vi "GetInstrumentInformation.vi"(8 "error in (no error)":errorcluster, 11 "RoomAlert in":refnum<class "RoomAlert.lvclass">) -> (0 "error out":errorcluster, 2 "Model IDs":string[][][](array[string]), 3 "RoomAlert out":refnum<class "RoomAlert.lvclass">)   [LabVIEW 2018, in "SensorPlugins.lvlib" / "RoomAlert.lvclass"]
doc: "Extracts the model name of the RoomAlert Instrument and also used to double check the connection to the instrument."
uses:
  RoomAlert.lvclass
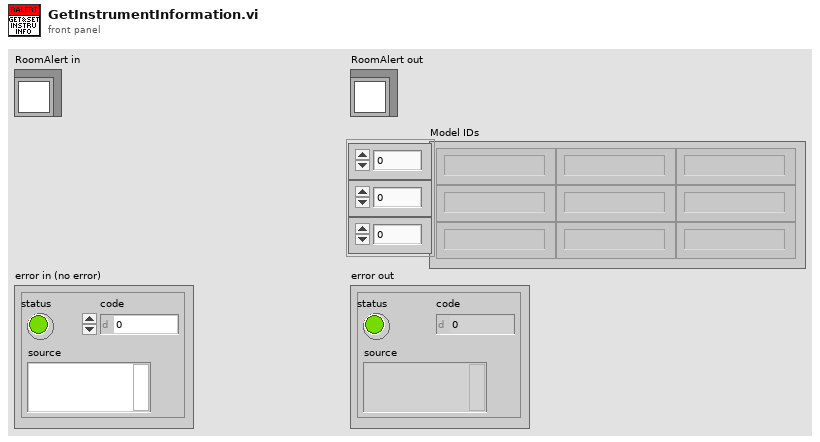
[diagram p1: front panel]
types:
  T1 = typedef "SensorPlugins.lvlib/RoomAlert.lvclass/RoomAlertControls.ctl" = cluster{"Connected?":bool, "IP Address of SNMP Device":string, "Port (161)":u16, "Community Name":string, "Measurements To Read Array":u16[], "Update LightTower?":bool, "LightTower":cluster{"Red":bool, "Amber":bool, "Green":bool, "Audio":bool}, "RoomAlert Model ID":string, "Sensor OID Numbers":string[][], "Sensor Light Tower OID Numbers":string[][]}[]
  T2 = typedef "SensorPlugins.lvlib/RoomAlert.lvclass/CommunicationControls.ctl" = refnum<k16>[]
  T3 = typedef "SensorPlugins.lvlib/RoomAlert.lvclass/MeasurementControls.ctl" = cluster{"Measurement RefreshTime (ms)":u32, "Measurement Name":string, "Timeout(ms)":i32, "Amber Warning Light Configuration":cluster{"Warning Temperture (Degrees C)":dbl, "Temperature Delta (Degrees C/Minute)":dbl, "Time Window (Minutes)":dbl}}
  T4 = cluster{"Connected?":bool, "IP Address of SNMP Device":string, "Port (161)":u16, "Community Name":string, "Measurements To Read Array":u16[], "Update LightTower?":bool, "LightTower":cluster{"Red":bool, "Amber":bool, "Green":bool, "Audio":bool}, "RoomAlert Model ID":string, "Sensor OID Numbers":string[][], "Sensor Light Tower OID Numbers":string[][]}
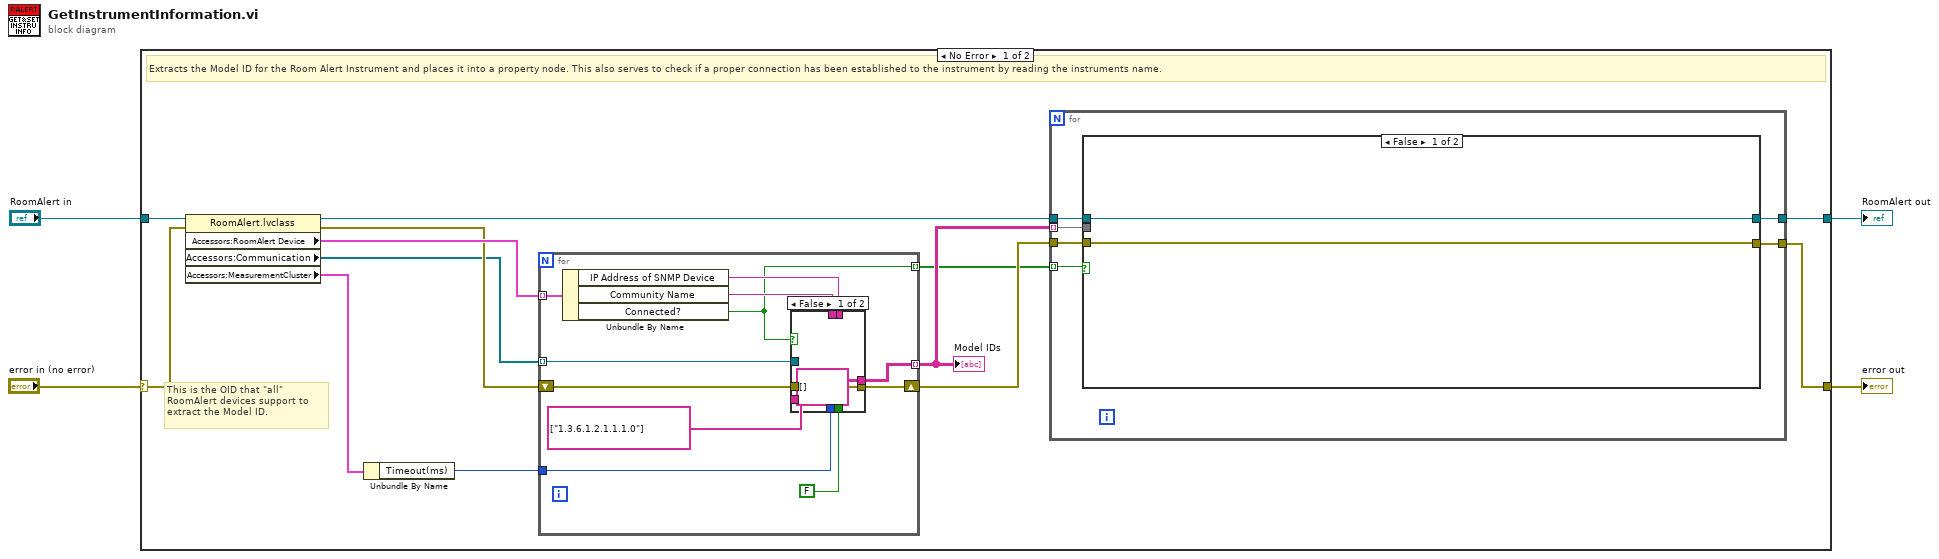
[diagram p0: block diagram]
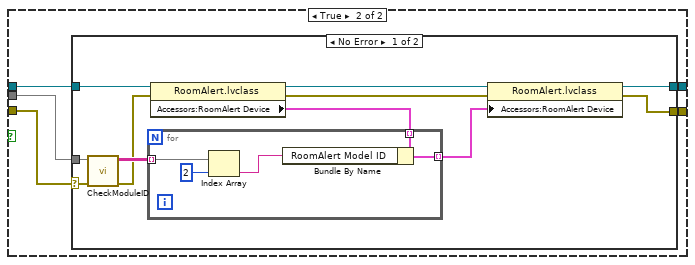
[diagram p2: hidden frame]
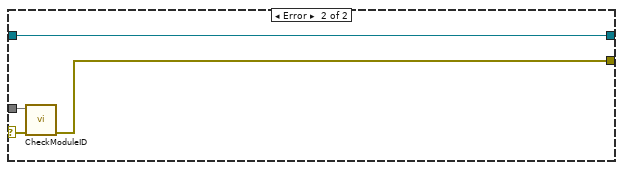
[diagram p3: hidden frame]
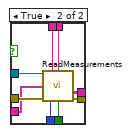
[diagram p4: hidden frame]
diagram:
  n1 = case shown="No Error" "error in (no error)" {
    selector: "error in (no error)" -> [w16 w74]
    tunnel: [w12 w74] -> w3
    tunnel: [w8 w73] -> w1
    tunnel: "RoomAlert in" -> [w17 w73]
    frame No Error {
      # "This is the OID that \"all\" \nRoomAlert devices support to \nextract the Model ID."
      # "Extracts the Model ID for the Room Alert Instrument and places it into a property node. This also serves to check if a proper connection has been established to the instrument by reading the instruments name."
      n2 = property class="RoomAlert.lvclass"(reference=w17, error in=w16) -> (reference out=w9:refnum<class "RoomAlert.lvclass">, error out=w14:errorcluster, "Accessors:RoomAlert Device"=w15:T1, "Accessors:Communication "=w13:T2, "Accessors:MeasurementCluster"=w7:T3)
      n3 = Unbundle By Name(w7) -> ("Timeout(ms)"=w6:i32)
      n4 = for {
        tunnel: w15 -> [w60] mode=indexing
        tunnel: w13 -> [w53] mode=indexing
        tunnel: [w54] -> w10 mode=indexing
        shift-right: [w61] -> w11
        shift-left: w14 -> [w59]
        tunnel: w6 -> [w52]
        tunnel: [w51] -> w5 mode=indexing
        n5 = Unbundle By Name(w60) -> ("IP Address of SNMP Device"=w58:string, "Community Name"=w57:string, "Connected?"=w51:bool)
        n6 = case shown="False" w51 {
          tunnel: [w63 w72] -> w61
          tunnel: w59 -> [w63 w71]
          tunnel: w58 -> [_ w70]
          tunnel: w57 -> [_ w69]
          tunnel: FALSE ("Filter OID Numbers? (T)") -> [_ w68]
          tunnel: string[] ["1.3.6.1.2.1.1.1.0"] -> [_ w67]
          tunnel: [string[][] [] ("SNMPDataAsStrings") w66] -> w54
          tunnel: w53 -> [_ w65]
          tunnel: w52 -> [_ w64]
          frame False {
          }
          frame True {
            n7 = call "ReadMeasurements.vi"("UDP Network Connection in"=w65, "Community Name"=w69, "IP Address of SNMP Device"=w70, "OID Numbers"=w67, "error in (no error)"=w71, "Timeout(ms)"=w64, "Filter OID Numbers? (T)"=w68) -> ("SNMPDataAsStrings"=w66:string[][], "error out"=w72:errorcluster)  [unwired: 5 in, 2 out]
          }
        }
      }
      "Model IDs" <- w10
      n8 = for {
        tunnel: w11 -> [w21]
        tunnel: [w22] -> w12
        tunnel: w9 -> [w23]
        tunnel: [w20] -> w8
        tunnel: w10 -> [w19] mode=indexing
        tunnel: w5 -> [w18] mode=indexing
        # "We check if a connection has actually been established"
        n9 = case shown="False" w18 {
          tunnel: w23 -> [w25 w30]
          tunnel: [w24 w29] -> w22
          tunnel: w21 -> [w24 w28]
          tunnel: [w25 w27] -> w20
          tunnel: w19 -> [_ w26]
          frame False {
          }
          frame True {
            n10 = case shown="No Error" w28 {
              selector: w28 -> [w33 w49]
              tunnel: w26 -> [w34 w48]
              tunnel: [w38 w47] -> w29
              tunnel: w30 -> [w41 w50]
              tunnel: [w39 w50] -> w27
              frame No Error {
                n11 = call "CheckModuleID.vi"("Error In"=w33, "Modle ID Array In"=w34) -> ("Error Out"=w31:errorcluster, "Modle ID ArrayOut"=w32:string[][])  [unwired: 8 in]
                n12 = property class="RoomAlert.lvclass"(reference=w41, error in=w31) -> (reference out=w40:refnum<class "RoomAlert.lvclass">, error out=w37:errorcluster, "Accessors:RoomAlert Device"=w36:T1)
                n13 = for {
                  tunnel: w36 -> [w46] mode=indexing
                  tunnel: w32 -> [w44] mode=indexing
                  tunnel: [w43] -> w35 mode=indexing
                  n14 = Index Array(array=w44, index=2 ("index (row)")) -> (element=w42:string)
                  n15 = Bundle By Name(cluster=w46, "RoomAlert Model ID"=w42) -> (w43:T4)
                }
                n16 = property class="RoomAlert.lvclass"(reference=w40, error in=w37, "Accessors:RoomAlert Device"=w35) -> (reference out=w39:refnum<class "RoomAlert.lvclass">, error out=w38:errorcluster)
              }
              frame Error {
                n17 = call "CheckModuleID.vi"("Error In"=w49, "Modle ID Array In"=w48) -> ("Error Out"=w47:errorcluster)  [unwired: 8 in, 1 out]
              }
            }
          }
        }
      }
    }
    frame Error {
    }
  }
  "error out" <- w3
  "RoomAlert out" <- w1
